vi "Read.vi"(6 "File Type":T1, 8 "error in (no error)":errorcluster, 11 "path":path) -> (0 "error out":errorcluster, 1 "Notes":string, 2 "Data (Dictionary)":T2[](array[typedef]), 3 "path out":path)   [LabVIEW 2016, in "Data.lvclass"]
uses:
  Data.lvclass
  Typedefs/Dictionary--cluster.ctl
  Typedefs/Type--enum.ctl
  Data.lvclass/Data.ctl
  Data.DAT/Data.DAT.lvclass
  C:/user/patrick/git/LV-to-ITX/src/Data/Data.lvclass
  Data.ITX/Data.ITX.lvclass
  Data.HDF5/Data.HDF5.lvclass
  Data.TDMS/Data.TDMS.lvclass
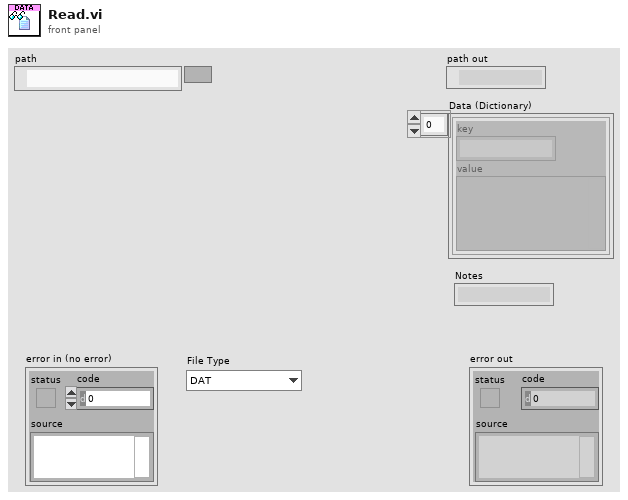
[diagram p1: front panel]
types:
  T1 = typedef "Data.lvclass/Type--enum.ctl" = enum16{"DAT", "ITX", "HDF5", "TDMS", "VI"}
  T2 = typedef "Data.lvclass/Dictionary--cluster.ctl" = cluster{"key":string, "value":variant}
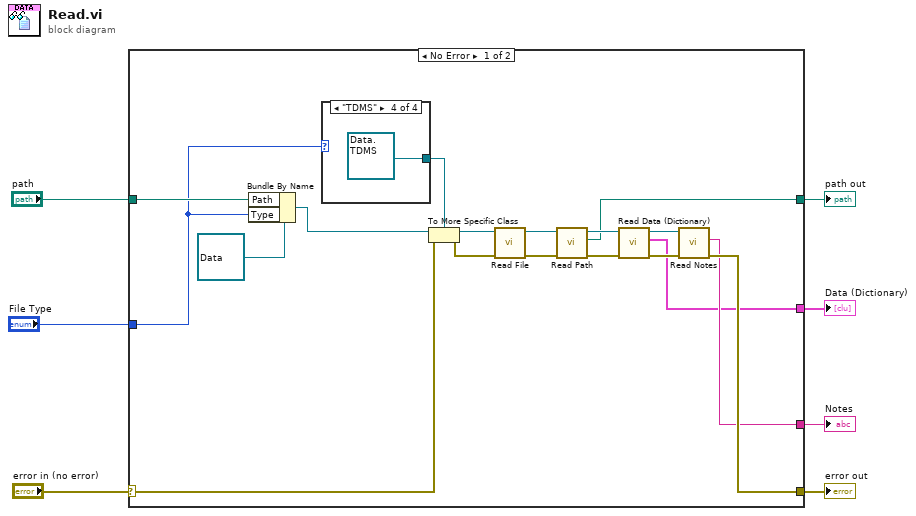
[diagram p0: block diagram]
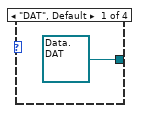
[diagram p2: hidden frame]
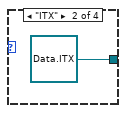
[diagram p3: hidden frame]
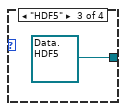
[diagram p4: hidden frame]
diagram:
  n1 = case shown="No Error" "error in (no error)" {
    selector: "error in (no error)" -> [w13 w31]
    tunnel: [w19 w31] -> w6
    tunnel: [w16 w30] -> w5
    tunnel: "path" -> [w12 w30]
    tunnel: "File Type" -> [w8 _]
    tunnel: [w17 _] -> w1
    tunnel: [w18 _] -> w2
    frame No Error {
      n2 = Bundle By Name(cluster=refnum<class "Data.lvclass"> refnum ("reference"), "Path"=w12, "Type"=w8) -> (w9:refnum<class "Data.lvclass">)
      n3 = case shown="\"TDMS\"" w8 {
        tunnel: [refnum<class "Data.DAT.lvclass"> refnum ("DAT.lvclass") refnum<class "Data.ITX.lvclass"> refnum ("ITX") refnum<class "Data.HDF5.lvclass"> refnum ("Data.HDF5.lvclass") refnum<class "Data.TDMS.lvclass"> refnum ("Data.TDMS.lvclass")] -> w15
        frame "DAT", Default {
        }
        frame "ITX" {
        }
        frame "HDF5" {
        }
        frame "TDMS" {
        }
      }
      n4 = To More Specific Class(target class=w15, reference=w9, error in=w13) -> (specific class reference=w11:refnum<class "Data.lvclass">, error out=w10:errorcluster)
      n5 = call-dynamic "Read File.vi"("error in (no error)"=w10, "Data Save in"=w11) -> ("error out"=w24:errorcluster, "Data Save out"=w25:refnum<class "Data.lvclass">)  [unwired: 8 in]
      n6 = call "Read Path.vi"("error in (no error)"=w24, "Data Save"=w25) -> ("error out"=w22:errorcluster, "Path"=w16:path, "Data Save out"=w23:refnum<class "Data.lvclass">)  [unwired: 7 in]
      n7 = call "Read Data (Dictionary).vi"("error in (no error)"=w22, "Data Save"=w23) -> ("error out"=w20:errorcluster, "Data (Dictionary)"=w17:T2[], "Data Save out"=w21:refnum<class "Data.lvclass">)  [unwired: 7 in]
      n8 = call "Read Notes.vi"("error in (no error)"=w20, "Data Save"=w21) -> ("error out"=w19:errorcluster, "Comments"=w18:string)  [unwired: 7 in, 1 out]
    }
    frame Error {
    }
  }
  "error out" <- w6
  "path out" <- w5
  "Data (Dictionary)" <- w1
  "Notes" <- w2
